vi "GetGXMLCfgDyn.vi"(8 "error in (no error)":errorcluster, 11 "Dynamic in":refnum<class "Dynamic.lvclass">) -> (0 "error out":errorcluster, 2 "DynChanCfg":T1, 3 "Dynamic out":refnum<class "Dynamic.lvclass">)   [LabVIEW 2018, in "Measurement Channels.lvlib" / "Dynamic.lvclass"]
uses:
  Dynamic.lvclass
  DynamicProps_TD.ctl
  Dynamic.lvclass/Dynamic.ctl
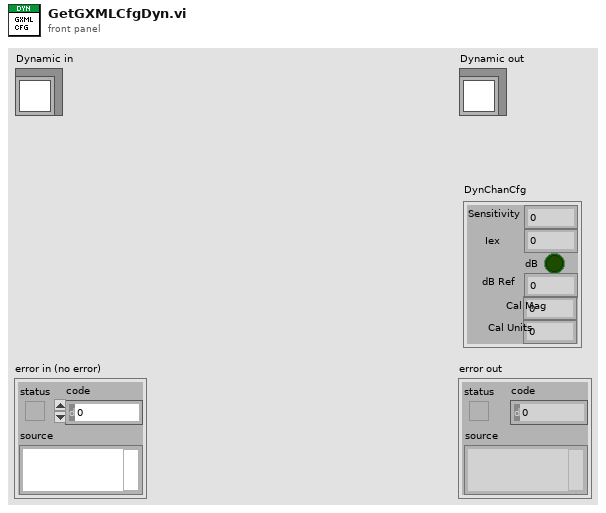
[diagram p1: front panel]
types:
  T1 = typedef "Measurement Channels.lvlib/Dynamic.lvclass/DynamicProps_TD.ctl" = cluster{"Sensitivity":dbl, "Iex":dbl, "dB":bool, "dB Ref":dbl, "Cal Mag":dbl, "Cal Units":u16}
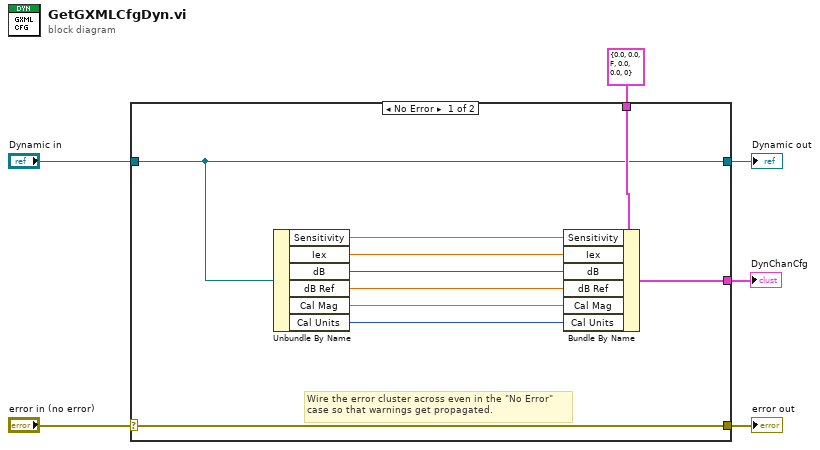
[diagram p0: block diagram]
diagram:
  n1 = case shown="No Error" "error in (no error)" {
    selector: "error in (no error)" -> [w16 w19]
    tunnel: [w16 w19] -> w5
    tunnel: [w14 w18] -> w3
    tunnel: "Dynamic in" -> [w14 w18]
    tunnel: T1 {"Sensitivity"=0.0, "Iex"=0.0, "dB"=FALSE, "dB Ref"=0.0, "Cal Mag"=0.0, "Cal Units"=0} ("DynChanCfg") -> [w15 w17]
    tunnel: [w7 w17] -> w1
    frame No Error {
      # "Wire the error cluster across even in the \"No Error\"\ncase so that warnings get propagated."
      n2 = Unbundle By Name(w14) -> ("Sensitivity"=w13:dbl, "Iex"=w12:dbl, "dB"=w11:bool, "dB Ref"=w10:dbl, "Cal Mag"=w9:dbl, "Cal Units"=w8:u16)
      n3 = Bundle By Name(cluster=w15, "Sensitivity"=w13, "Iex"=w12, "dB"=w11, "dB Ref"=w10, "Cal Mag"=w9, "Cal Units"=w8) -> (w7:T1)
    }
    frame Error {
    }
  }
  "error out" <- w5
  "Dynamic out" <- w3
  "DynChanCfg" <- w1
